vi "RT_Propulsive_Moment_in_DLR_Navigation_Reference_System_2 (SubVI).vi"(5 "FE":dbl[](array[numeric]), 8 "Vehicle Parameters":T2, 9 "Rotation":T1, 10 "i":i32, 11 "Data":dbl[][](array[numeric])) -> (3 "MFE (Nm)":dbl[](array[numeric]))   [LabVIEW 2017]
uses:
  <vilib>/Analysis/baseanly.llb/Real A x B.vi
  <vilib>/Analysis/Matrix/Numeric/Conversions/Array To Matrix - RA.vi
  <vilib>/Analysis/Matrix/Numeric/Conversions/Array To Matrix - RA2.vi
  <vilib>/Analysis/Matrix/Numeric/Conversions/Matrix To Array - RM.vi
  <vilib>/Analysis/NI_AALBase.lvlib
  <vilib>/Analysis/Matrix/NI_Matrix.lvlib
  <vilib>/Analysis/NI_AALPro.lvlib
panel:
  out "Re":dbl[](array[numeric])
  out "re":dbl
  out "CoG (m)":dbl
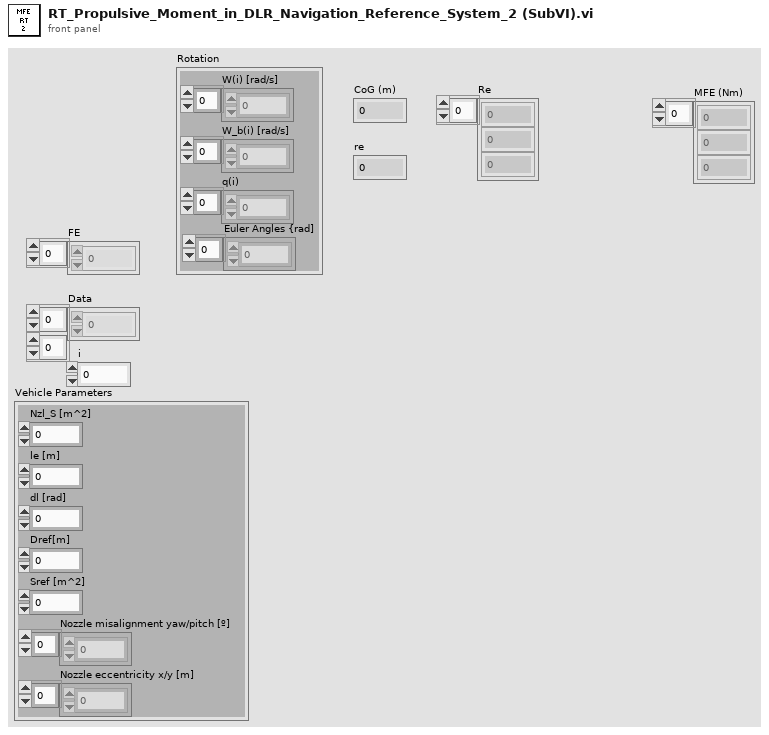
[diagram p1: front panel]
types:
  T1 = cluster{"W(i) [rad/s]":dbl[], "W_b(i) [rad/s]":dbl[], "q(i)":dbl[], "Euler Angles {rad]":dbl[]}
  T2 = cluster{"Nzl_S [m^2]":dbl, "le [m]":dbl, "dl [rad]":dbl, "Dref[m]":dbl, "Sref [m^2]":dbl, "Nozzle misalignment yaw/pitch [º]":dbl[], "Nozzle eccentricity x/y [m]":dbl[]}
  T3 = typedef "NI_Matrix.lvlib/RealMatrix.ctl" = dbl[][]
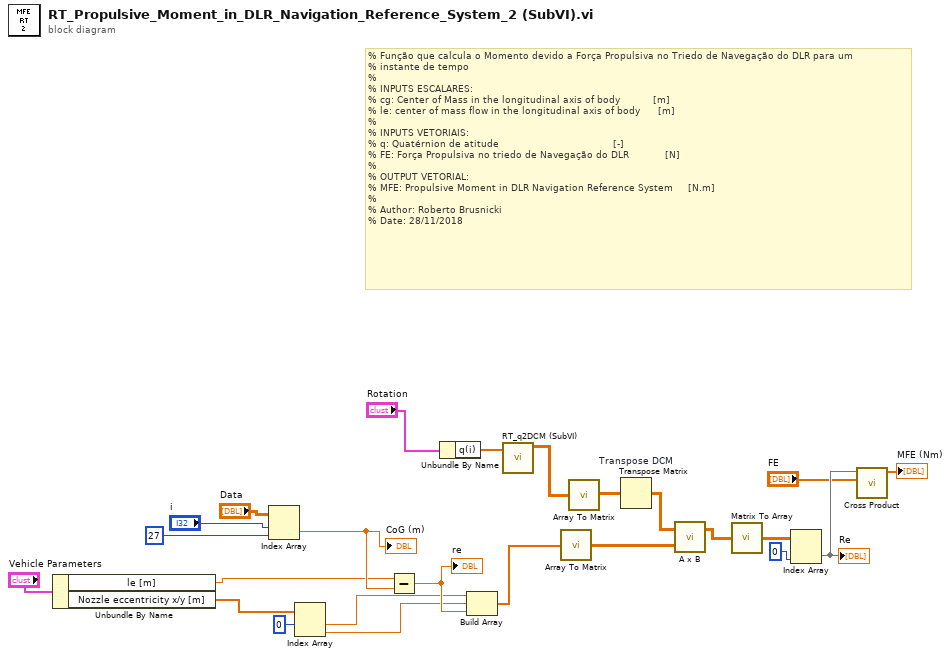
[diagram p0: block diagram]
diagram:
  # "% Função que calcula o Momento devido a Força Propulsiva no Triedo de Navegação do DLR para um \n% instante de tempo\n%\n% INPUTS ESCALARES:\n% cg: Center of Mass in the longitudinal axis of body           [m]\n% le: center of mass flow in the longitudinal axis of body      [m]\n% \n% INPUTS VETORIAIS:\n% q: Quatérnion de atitude                                      [-]\n% FE: Força Propulsiva no triedo de Navegação do DLR            [N] \t\n%\n% OUTPUT VETORIAL:\n% MFE: Propulsive Moment in DLR Navigation Reference System     [N.m]\n%\n% Author: Roberto Brusnicki\n% Date: 28/11/2018"
  n1 = Unbundle By Name("Vehicle Parameters") -> ("le [m]"=w9:dbl, "Nozzle eccentricity x/y [m]"=w4:dbl[])
  n2 = Index Array(array="Data", index (row)="i", index (col)=27 ("disabled index (col)")) -> (element=w21:dbl)
  "CoG (m)" <- w21
  n3 = Index Array(array=w4, index #1=0 ("index")) -> (element #1=w8:dbl, element #2=w7:dbl)  [unwired: 1 in]
  n4 = Subtract(x=w9, y=w21) -> (x-y=w17:dbl)
  "re" <- w17
  n5 = Unbundle By Name("Rotation") -> ("q(i)"=w3:dbl[])
  n6 = Build Array(w8, w7, w17) -> (w18:dbl[])
  n7 = call "RT_q2DCM (SubVI).vi"("Quaternion"=w3) -> ("DCM"=w2:dbl[][])  [unwired: 10 in]
  n8 = call-poly <vilib>:"Array To Matrix.vi"("Real 1D Array"=w18) -> ("Real Matrix (Column Vector)"=w16:T3)
  n9 = call-poly <vilib>:"Array To Matrix.vi"("Real 2D Array"=w2) -> ("Real Matrix"=w19:T3)
  n10 = Transpose Matrix "Transpose DCM"(1:w19) -> (0:w20:T3)
  n11 = call-poly <vilib>:"A x B.vi"("B"=w16, "A"=w20) -> ("A x B"=w14:T3)  [unwired: 1 out]
  n12 = call-poly <vilib>:"Matrix To Array.vi"("Real Matrix"=w14) -> ("Real 2D Array"=w15:dbl[][])
  n13 = Index Array(array=w15, index (col)=0 ("index (row)")) -> (element=w23:dbl[])  [unwired: 1 in]
  "Re" <- w23
  n14 = call <vilib>:"Cross Product.vi"("B Vector"="FE", "A Vector"=w23) -> ("Cross Product"=→"MFE (Nm)":dbl[])  [unwired: 8 in, 1 out]
